vi "GV_YscaleCalcScaleSpecs.vi"(0 "FormatString":string="%_3f", 1 "desired font(Application)":T4(ring)=enum."Application Font", 2 "scale definition":T1={"coordinate 1"=5, "value 1"=5.0, "coordinate 2"=5, "value 2"=5.0, "log?(F)"=FALSE} {"value 2" format="%0.2f"; "value 1" format="%0.2f"}, 3 "scale attributes":T2={"horizontal"=TRUE, "left/top"=FALSE, "draw bar"=FALSE, "line color"=0, "text color(black)"=0}, 5 "[user-specified font]":T3) -> (7 "scale specs":cluster{"coordinate":i16, "label":string}[](array[cluster])=[{"coordinate"=7, "label"="1"}, {"coordinate"=23, "label"="2"}])   [LabVIEW 2020, in "Sgraph_lib_V1.lvlib" / "Gviewer.lvclass"]
doc: "Source: NI LV13\nTakes a specification for a Cartesian style scale and calculates the coordinates and labels to use for the scale.\n---------------------------------------------------------------\nAndre Koelewijn, 12 sept 2014 Rev 2:\nAdapted the code for use with the DCS historian graph display."
uses:
  Gviewer.lvclass
  Gviewer.lvclass/Gviewer.ctl
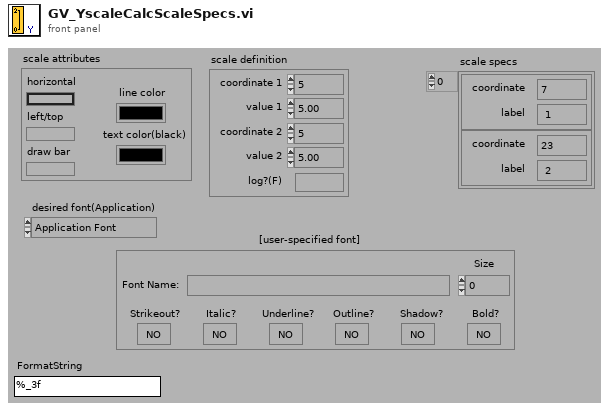
[diagram p1: front panel]
types:
  T1 = cluster{"coordinate 1":i16, "value 1":dbl, "coordinate 2":i16, "value 2":dbl, "log?(F)":bool}
  T2 = cluster{"horizontal":bool, "left/top":bool, "draw bar":bool, "line color":u32, "text color(black)":u32}
  T3 = cluster{"Font Name:":string, "Size":i16, "Strikeout?":bool, "Italic?":bool, "Underline?":bool, "Outline?":bool, "Shadow?":bool, "Bold?":bool}
  T4 = enum16{"User-specified Font", "Application Font", "System Font", "Dialog Font"}
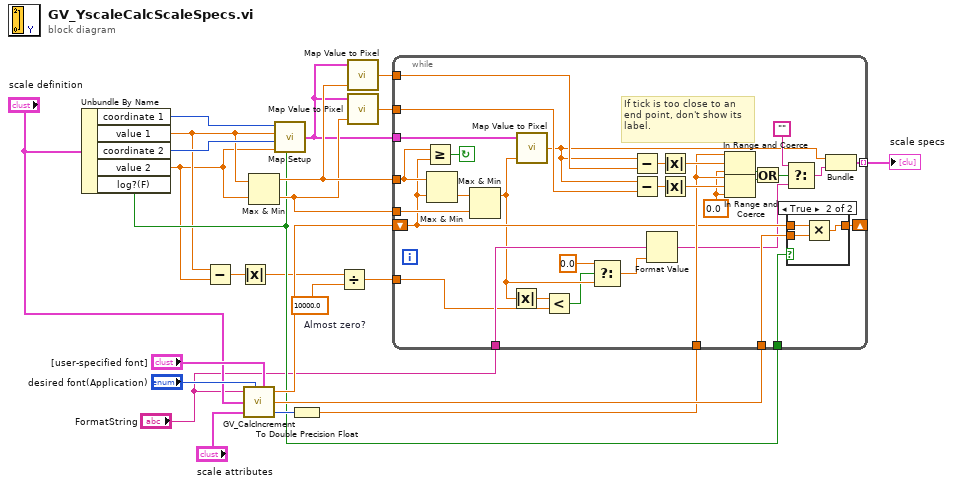
[diagram p0: block diagram]
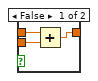
[diagram p2: hidden frame]
diagram:
  w2 = 10000.0  # Almost zero?
  n1 = Unbundle By Name("scale definition") -> ("coordinate 1"=w19:i16, "value 1"=w6:dbl, "coordinate 2"=w23:i16, "value 2"=w5:dbl, "log?(F)"=w10:bool)
  n2 = Subtract(x=w6, y=w5) -> (x-y=w4:dbl)
  n3 = Absolute Value(x=w4) -> (abs(x)=w3:dbl)
  n4 = call "GV_CalcIncrement.vi"("FormatString"="FormatString", "desired font(Application)"="desired font(Application)", "scale definition"="scale definition", "scale attributes"="scale attributes", "[user-specified font]"="[user-specified font]") -> ("start"=w12:dbl, "increment"=w24:dbl, "text size"=w22:i16)  [unwired: 2 in]
  n5 = Max & Min(x=w6, y=w5) -> (max(x,y)=w21:dbl, min(x,y)=w20:dbl)
  n6 = call <vilib>:"Map Setup.vi"("coordinate 1"=w19, "value 1"=w6, "coordinate 2"=w23, "value 2"=w5, "log?(F)"=w10) -> ("scale factors"=w18:cluster{"a":dbl, "b":dbl, "log?(F)":bool})
  n7 = To Double Precision Float(number=w22) -> (double precision float=w9:dbl)
  n8 = Divide(x=w3, y=w2) -> (x/y=w1:dbl)
  n9 = call <vilib>:"Map Value to Pixel.vi"("x"=w21, "scale factors"=w18) -> ("pixel"=w17:dbl)  [unwired: 1 in]
  n10 = call <vilib>:"Map Value to Pixel.vi"("x"=w20, "scale factors"=w18) -> ("pixel"=w16:dbl)  [unwired: 1 in]
  n11 = while {
    tunnel: w10 -> [w33]
    tunnel: w16 -> [w43]
    tunnel: w17 -> [w50]
    tunnel: w9 -> [w42]
    tunnel: [w55] -> w11 mode=indexing
    tunnel: w24 -> [w36]
    tunnel: w18 -> [w51]
    tunnel: w20 -> [w53]
    tunnel: w21 -> [w52]
    shift-left: w12 -> [w35]
    shift-right: [w34] -> _
    tunnel: "FormatString" -> [w31]
    tunnel: w1 -> [w26]
    stop <- w54 continue-if-true
    w41 = 0.0
    # "If tick is too close to an\nend point, don't show its\nlabel."
    n12 = Greater Or Equal?(x=w52, y=w35) -> (x >= y?=w54:bool)
    n13 = Max & Min(x=w52, y=w35) -> (min(x,y)=w56:dbl)  [unwired: 1 out]
    n14 = Max & Min(x=w56, y=w53) -> (max(x,y)=w28:dbl)  [unwired: 1 out]
    n15 = Absolute Value(x=w28) -> (abs(x)=w27:dbl)
    n16 = call <vilib>:"Map Value to Pixel.vi"("x"=w28, "scale factors"=w51) -> ("pixel"=w37:dbl)  [unwired: 1 in]
    n17 = Less?(x=w27, y=w26) -> (x < y?=w25:bool)
    n18 = Select(t=0.0, s=w25, f=w28) -> (s? t:f=w30:dbl)
    n19 = Subtract(x=w37, y=w50) -> (x-y=w49:dbl)
    n20 = Subtract(x=w37, y=w43) -> (x-y=w44:dbl)
    n21 = Format Value(format string=w31, value (0)=w30) -> (output string=w32:string)  [unwired: 1 in]
    n22 = Absolute Value(x=w49) -> (abs(x)=w48:dbl)
    n23 = Absolute Value(x=w44) -> (abs(x)=w45:dbl)
    n24 = In Range and Coerce(upper limit=w42, x=w48, lower limit=w41) -> (In Range?=w39:bool)  [unwired: 1 out]
    n25 = In Range and Coerce(upper limit=w42, x=w45, lower limit=w41) -> (In Range?=w38:bool)  [unwired: 1 out]
    n26 = Or(x=w39, y=w38) -> (x .or. y?=w40:bool)
    n27 = Select(t="", s=w40, f=w32) -> (s? t:f=w46:string)
    n28 = case shown="True" w33 {
      tunnel: w36 -> [w58 w62]
      tunnel: w35 -> [w57 w61]
      tunnel: [w59 w60] -> w34
      frame False {
        n29 = Add(x=w57, y=w58) -> (x+y=w59:dbl)
      }
      frame True {
        n30 = Multiply(x=w61, y=w62) -> (x*y=w60:dbl)
      }
    }
    n31 = Bundle("pixel"=w37, "output string"=w46) -> (w55:cluster{"pixel":dbl, "output string":string})  [unwired: 1 in]
  }
  "scale specs" <- w11
